vi "init data cluster.vi"(0 "data clusters in":T2[](array[typedef]), 5 "shared memory name":string, 7 "channel classification":T3, 9 "data type":T1, 11 "error in (no error)":errorcluster, 12 "index":i32) -> (4 "data clusters out":T2[](array[typedef]), 15 "error out":errorcluster)   [LabVIEW 2013, in "Shared Memory runtime.lvclass"]
uses:
  Shared Memory runtime.lvclass
  <vilib>/NI/Tag Bus Module Framework/channel/channel classification.ctl
  channel runtime.ctl
  <vilib>/NI/Tag Bus/tag/Data Type.ctl
  <vilib>/NI/Shared Memory Library/Classes/Shared Memory/Public/Controls/reference.ctl
  <vilib>/NI/Shared Memory Library/Classes/Shared Memory/Shared Memory.lvclass
  <vilib>/NI/Shared Memory Library/Classes/Shared Memory/Public/Controls/file mode.ctl
  <vilib>/NI/Shared Memory Library/Classes/Shared Memory/Public/Controls/permissions group.ctl
  <vilib>/NI/Shared Memory Library/Classes/Shared Memory/Public/Controls/permissions.ctl
  <vilib>/NI/Tag Bus/tag/tag descriptor.lvclass
  <vilib>/NI/Tag Bus Module Framework/channel/TBM channel.lvclass
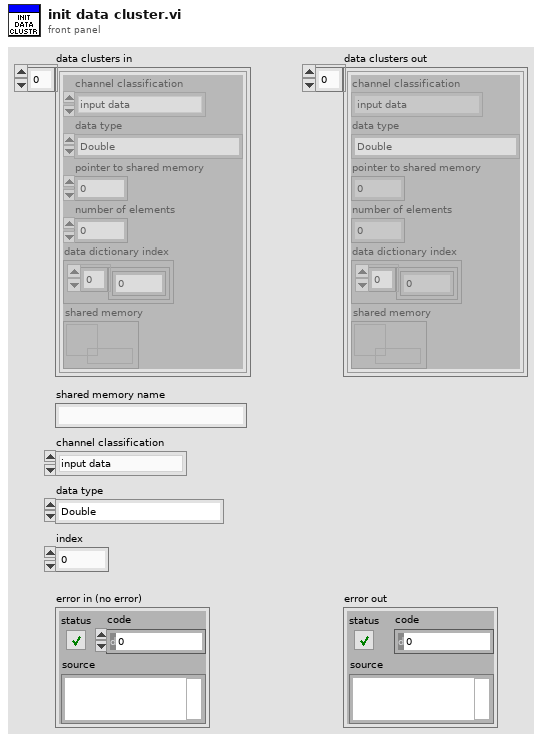
[diagram p1: front panel]
types:
  T1 = typedef "tag bus.lvlib/tag descriptor.lvclass/Data Type.ctl" = enum16{"Double", "Single", "I64", "I32", "I16", "I8", "U64", "U32", "U16", "U8", "Boolean", "String", "Array of Double", "Array of Single", "Array of I64", "Array of I32", "Array of I16", "Array of I8", "Array of U64", "Array of U32", "Array of U16", "Array of U8", "Array of Boolean", "Array of String"}
  T2 = typedef "Shared Memory runtime.lvclass/channel runtime.ctl" = cluster{"channel classification":T3, "data type":T1, "pointer to shared memory":u64, "number of elements":u64, "data dictionary index":cluster{i32[]}, "shared memory":T4}
  T3 = typedef "TBM channel.lvclass/channel classification.ctl" = enum16{"input data", "output data", "processing parameter", "processing result"}
  T4 = typedef "Shared Memory.lvlib/Shared Memory.lvclass/reference.ctl" = refnum<data-value>
  T5 = typedef "Shared Memory.lvlib/Shared Memory.lvclass/permissions group.ctl" = cluster{"owner":T6, "group":T6, "everyone":T6}
  T6 = typedef "Shared Memory.lvlib/Shared Memory.lvclass/permissions.ctl" = cluster{"read":bool, "write":bool, "execute":bool}
  T7 = typedef "Shared Memory.lvlib/Shared Memory.lvclass/file mode.ctl" = enum16{"open", "create/replace"}
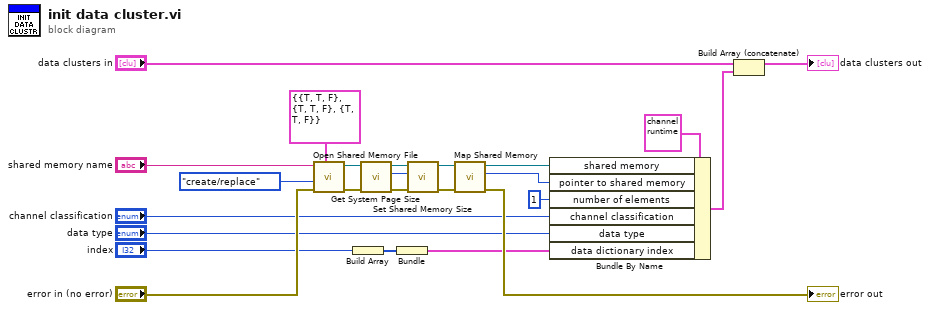
[diagram p0: block diagram]
diagram:
  n1 = call <vilib>:"Open Shared Memory File.vi"("permissions (0664)"=T5 {"owner"={"read"=TRUE, "write"=TRUE, "execute"=FALSE}, "group"={"read"=TRUE, "write"=TRUE, "execute"=FALSE}, "everyone"={"read"=TRUE, "write"=TRUE, "execute"=FALSE}}, "error in (no error)"="error in (no error)", "file mode (open)"=file_mode."create/replace" ("file mode (default: open)"), "shared memory name"="shared memory name") -> ("error out"=w12:errorcluster, "shared memory out"=w8:T4)  [unwired: 6 in]
  n2 = Build Array("index") -> (w18:i32[])
  n3 = call <vilib>:"Get System Page Size.vi"("error in (no error)"=w12, "shared memory in"=w8) -> ("error out"=w13:errorcluster, "page size (bytes)"=w11:u32, "shared memory out"=w9:T4)  [unwired: 7 in]
  n4 = Bundle(w18) -> (w20:cluster{i32[]})  [unwired: 1 in]
  n5 = call <vilib>:"Set Shared Memory Size.vi"("error in (no error)"=w13, "size (bytes)"=w11, "shared memory in"=w9) -> ("error out"=w14:errorcluster, "shared memory out"=w10:T4)  [unwired: 7 in]
  n6 = call <vilib>:"Map Shared Memory.vi"("error in (no error)"=w14, "shared memory in"=w10) -> ("error out"=→"error out":errorcluster, "pointer to shared memory"=w16:u64, "shared memory out"=w22:T4)  [unwired: 7 in]
  n7 = Bundle By Name(cluster=T2 {"channel classification"=enum."input data", "data type"=enum."Double", "pointer to shared memory"=0, "number of elements"=0, "data dictionary index"={[]}, "shared memory"=refnum} ("runtime"), "shared memory"=w22, "pointer to shared memory"=w16, "number of elements"=u64 1 ("quantity"), "channel classification"="channel classification", "data type"="data type", "data dictionary index"=w20) -> (w5:T2)
  n8 = Build Array (concatenate)("data clusters in", w5) -> (→"data clusters out":T2[])
